vi "readFromXML.vi"(8 "error in (no error)":errorcluster, 10 "XML in":string, 11 "AbsorbPOrigin in":refnum<class "AbsorbPOrigin.lvclass">) -> (0 "error out":errorcluster, 3 "AbsorbPOrigin out":refnum<class "AbsorbPOrigin.lvclass">)   [LabVIEW 2022 SP3, in "TCSDataDefinitions.lvlib" / "TCSCommand.lvlib" / "POriginCommands.lvlib" / "AbsorbPOrigin.lvclass"]
uses:
  AbsorbPOrigin.lvclass
  OffsetCommands/Enumerations/Num2Types.ctl
  AbsorbPOrigin.lvclass/AbsorbPOrigin.ctl
  POriginCommands/POriginCommands.lvclass
  <userlib>/Common/XML/XMLParser/XMLParser.lvclass
  OffsetCommands/OffsetCommands.lvlib
panel:
  out "num2":T1
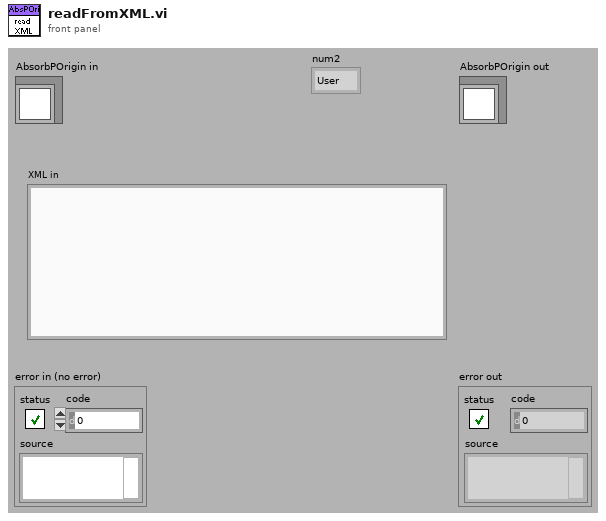
[diagram p1: front panel]
types:
  T1 = typedef "TCSDataDefinitions.lvlib/TCSCommand.lvlib/OffsetCommands.lvlib/Num2Types.ctl" = enum16{"User", "Handset", "Both"}
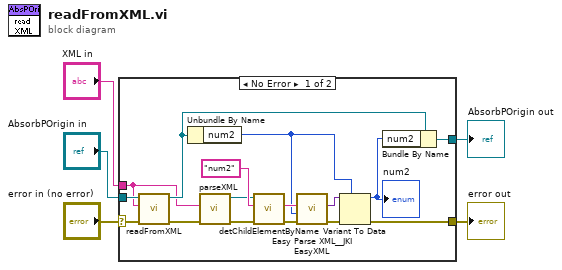
[diagram p0: block diagram]
diagram:
  n1 = case shown="No Error" "error in (no error)" {
    selector: "error in (no error)" -> [w16 w23]
    tunnel: [w9 w23] -> w4
    tunnel: [w19 w22] -> w2
    tunnel: "AbsorbPOrigin in" -> [w18 w22]
    tunnel: "XML in" -> [w14 _]
    frame No Error {
      n2 = call-parent "readFromXML.vi"("error in (no error)"=w16, "XML in"=w14, "POriginCommands in"=w18) -> ("error out"=w15:errorcluster, "POriginCommands out"=w17:refnum<class "AbsorbPOrigin.lvclass">)  [unwired: 7 out]
      n3 = Unbundle By Name(w17) -> ("num2"=w8:T1)
      n4 = call <userlib>:"parseXML.vi"("error in (no error)"=w15, "XMLString in"=w14) -> ("error out"=w20:errorcluster, "Element out"=w6:refnum<class "XMLParser.lvclass">)  [unwired: 8 in]
      n5 = call <userlib>:"detChildElementByName.vi"("error in (no error)"=w20, "childName"="num2" ("ChildName"), "Element in"=w6) -> ("error out"=w10:errorcluster, "childXML"=w11:string)  [unwired: 5 in, 2 out]
      n6 = call <vilib>:"Easy Parse XML__JKI EasyXML.vi"("error in (no error)"=w10, "LabVIEW Data (Type)"=w8, "XML String"=w11) -> ("error out"=w13:errorcluster, "LabVIEW Data"=w12:variant)  [unwired: 7 in]
      n7 = Variant To Data(error in=w13, type=w8, Variant=w12) -> (data=w7:T1, error out=w9:errorcluster)
      "num2" <- w7
      n8 = Bundle By Name(cluster=w17, "num2"=w7) -> (w19:refnum<class "AbsorbPOrigin.lvclass">)
    }
    frame Error {
    }
  }
  "error out" <- w4
  "AbsorbPOrigin out" <- w2
